vi "NanonisProperties_troubleshooting.vi"(1 "Z Write (m)":sgl format="%#_6p", 5 "X pen (nm)":dbl, 7 "Y pen (nm)":dbl, 12 "Z Write?":bool) -> (2 "Frame Size (m)":cluster{"Width":sgl, "Height":sgl} {"Height" format="%.2p"; "Width" format="%.2p"}, 3 "Frame Origin (m)":cluster{"Xc":sgl, "Yc":sgl} {"Yc" format="%.2p"; "Xc" format="%.2p"}, 8 "Current (pA)":sgl format="%#_6p", 10 "Z Read (m)":sgl format="%#_6p")   [LabVIEW 2019]
uses:
  <userlib>/Nanonis Prog Interface V5/Nanonis Prog Interface.lvlib
panel:
  in  "Manual Safetip":bool
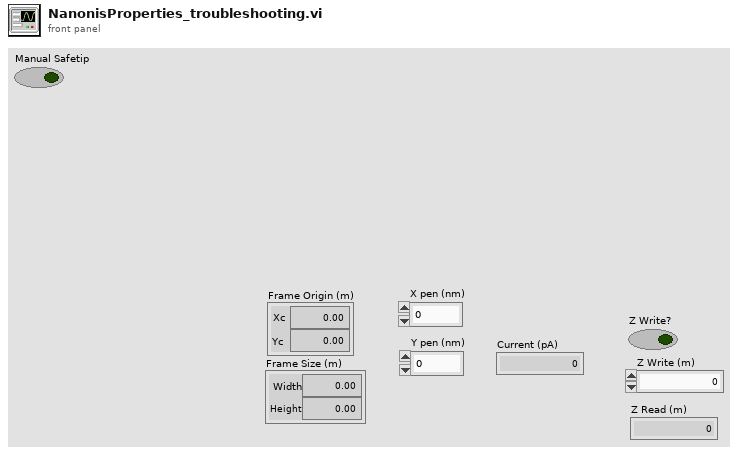
[diagram p1: front panel]
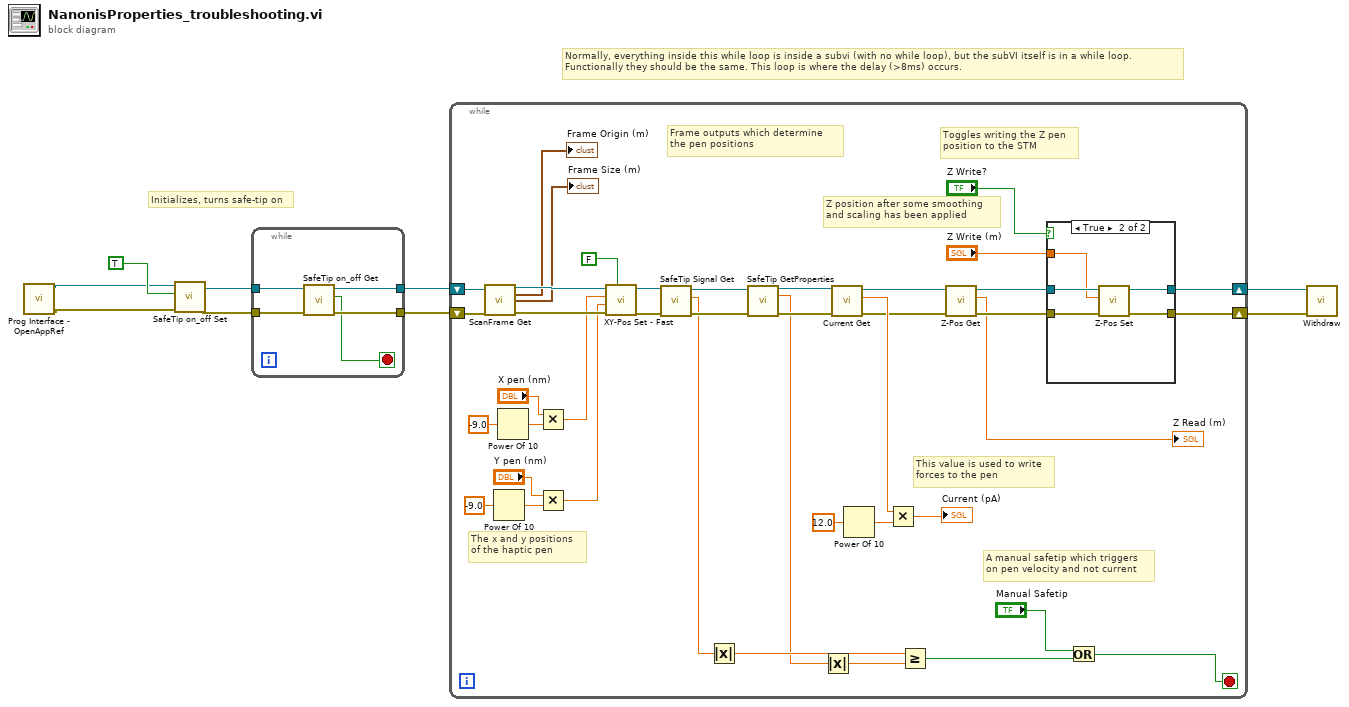
[diagram p0: block diagram]
diagram:
  # "Normally, everything inside this while loop is inside a subvi (with no while loop), but the subVI itself is in a while loop.\nFunctionally they should be the same. This loop is where the delay (>8ms) occurs."
  # "Initializes, turns safe-tip on"
  n1 = call <userlib>:"Prog Interface - OpenAppRef.vi"() -> ("Error out"=w7:errorcluster, "Application reference"=w8:refnum<vi>)  [unwired: 6 in]
  n2 = call <userlib>:"SafeTip on_off Set.vi"("error in (no error)"=w7, "SafeTip ON/OFF"=TRUE, "Application ref in"=w8) -> ("error out"=w5:errorcluster, "Application ref out"=w6:refnum<vi>)  [unwired: 7 in]
  n3 = while {
    tunnel: w6 -> [w14]
    tunnel: w5 -> [w13]
    tunnel: [w12] -> w4
    tunnel: [w11] -> w3
    stop <- w10 stop-if-true
    n4 = call <userlib>:"SafeTip on_off Get.vi"("error in (no error)"=w13, "Application ref in"=w14) -> ("error out"=w12:errorcluster, "SafeTip on/off status"=w10:bool, "Application ref out"=w11:refnum<vi>)  [unwired: 7 in]
  }
  n5 = while {
    shift-right: [w32] -> w1
    shift-left: w3 -> [w54]
    shift-right: [w31] -> w2
    shift-left: w4 -> [w53]
    stop <- w16 stop-if-true
    # "Frame outputs which determine \nthe pen positions"
    # "Z position after some smoothing\nand scaling has been applied"
    # "Toggles writing the Z pen\nposition to the STM"
    # "This value is used to write \nforces to the pen"
    # "A manual safetip which triggers\non pen velocity and not current"
    # "The x and y positions \nof the haptic pen"
    n6 = call <userlib>:"ScanFrame Get.vi"("Application ref in"=w54, "error in (no error)"=w53) -> ("Application ref out"=w52:refnum<vi>, "Center coordinates (m)"=→"Frame Origin (m)":cluster{"Xc":sgl, "Yc":sgl}, "Size (m)"=→"Frame Size (m)":cluster{"Width":sgl, "Height":sgl}, "error out"=w51:errorcluster)  [unwired: 9 in, 1 out]
    n7 = Power Of 10(x=-9.0) -> (10^x=w45:dbl)
    n8 = Power Of 10(x=-9.0) -> (10^x=w48:dbl)
    n9 = Multiply(x="X pen (nm)", y=w48) -> (x*y=w42:dbl)
    n10 = Multiply(x="Y pen (nm)", y=w45) -> (x*y=w41:dbl)
    n11 = call <userlib>:"XY-Pos Set - Fast.vi"("Wait end-of-motion (T=True)"=FALSE, "error in (no error)"=w51, "Y (m)"=w41, "X (m)"=w42, "Application ref in"=w52) -> ("error out"=w26:errorcluster, "Application ref out"=w27:refnum<vi>)  [unwired: 4 in]
    n12 = call <userlib>:"SafeTip Signal Get.vi"("error in (no error)"=w26, "Application ref in"=w27) -> ("error out"=w22:errorcluster, "SafeTip signal value"=w21:sgl, "Application ref out"=w25:refnum<vi>)  [unwired: 7 in]
    n13 = Absolute Value(x=w21) -> (abs(x)=w20:sgl)
    n14 = call <userlib>:"SafeTip GetProperties.vi"("Application ref in"=w25, "error in (no error)"=w22) -> ("Application ref out"=w24:refnum<vi>, "Threshold"=w19:sgl, "error out"=w23:errorcluster)  [unwired: 9 in, 2 out]
    n15 = Absolute Value(x=w19) -> (abs(x)=w18:sgl)
    n16 = call <userlib>:"Current Get.vi"("Error in (no error)"=w23, "Application ref in"=w24) -> ("Error out"=w35:errorcluster, "Current (A)"=w37:sgl, "Application ref out"=w36:refnum<vi>)  [unwired: 5 in]
    n17 = Power Of 10(x=12.0) -> (10^x=w38:dbl)
    n18 = Multiply(x=w37, y=w38) -> (x*y=→"Current (pA)":dbl)
    n19 = Greater Or Equal?(x=w20, y=w18) -> (x >= y?=w17:bool)
    n20 = call <userlib>:"Z-Pos Get.vi"("error in (no error)"=w35, "Application ref in"=w36) -> ("error out"=w33:errorcluster, "Z position (m)"=→"Z Read (m)":sgl, "Application ref out"=w34:refnum<vi>)  [unwired: 7 in]
    n21 = case shown="True" "Z Write?" {
      tunnel: w34 -> [w57 w62]
      tunnel: w33 -> [w56 w61]
      tunnel: [w57 w60] -> w32
      tunnel: [w56 w59] -> w31
      tunnel: "Z Write (m)" -> [_ w58]
      frame False {
      }
      frame True {
        n22 = call <userlib>:"Z-Pos Set.vi"("error in (no error)"=w61, "Z position (m)"=w58, "Application ref in"=w62) -> ("error out"=w59:errorcluster, "Application ref out"=w60:refnum<vi>)  [unwired: 7 in]
      }
    }
    n23 = Or(x="Manual Safetip", y=w17) -> (x .or. y?=w16:bool)
  }
  n24 = call <userlib>:"Withdraw.vi"("Error in (no error)"=w2, "Application ref in"=w1) -> ()  [unwired: 8 in, 2 out]
